vi "emi_int Changed.vi"(7 "x":i32) -> (6 "Rising":bool, 8 "changed":bool, 10 "Falling":bool)   [LabVIEW 2010]
doc: "Monitors a int 32, indicateing change, and wheter it was rising or falling. \n\nOn first call, it uses the input as previous as well, returning false.\n\nreentrant Subroutine."
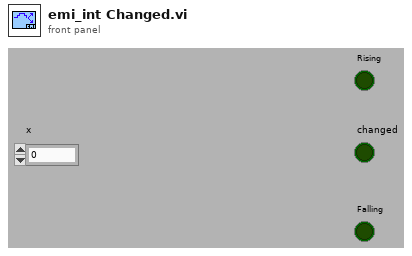
[diagram p1: front panel]
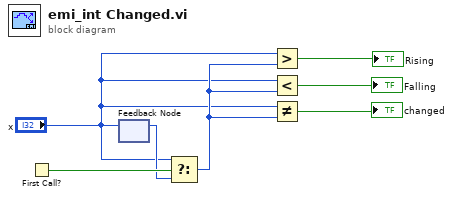
[diagram p0: block diagram]
diagram:
  n1 = First Call?() -> (First Call?: T/F=w7:bool)
  n2 = feedback-in #1("x") -> ()
  n3 = feedback #1() -> (w5:i32)  [unwired: 1 in]
  n4 = Select(t="x", s=w7, f=w5) -> (s? t:f=w4:i32)
  n5 = Greater?(x="x", y=w4) -> (0:→"Rising":bool)
  n6 = Less?(x="x", y=w4) -> (x < y?=→"Falling":bool)
  n7 = Not Equal?(x="x", y=w4) -> (x != y?=→"changed":bool)
